vi "FTW-TransferClient-Destroy.vi"(0 "TransferClient.dotNET":refnum<class "FTW-TransferClient-dotNET.lvclass">, 11 "error in":errorcluster) -> (15 "error out":errorcluster)   [LabVIEW 2012, in "FTW-TransferClient-dotNET.lvclass"]
uses:
  FTW-TransferClient-dotNET.lvclass
  FTW-TransferClient.lvclass
  FTW-TransferClient-dotNET.lvclass/FTW-TransferClient-dotNET.ctl
panel:
  # "Inputs"
  # "Outputs"
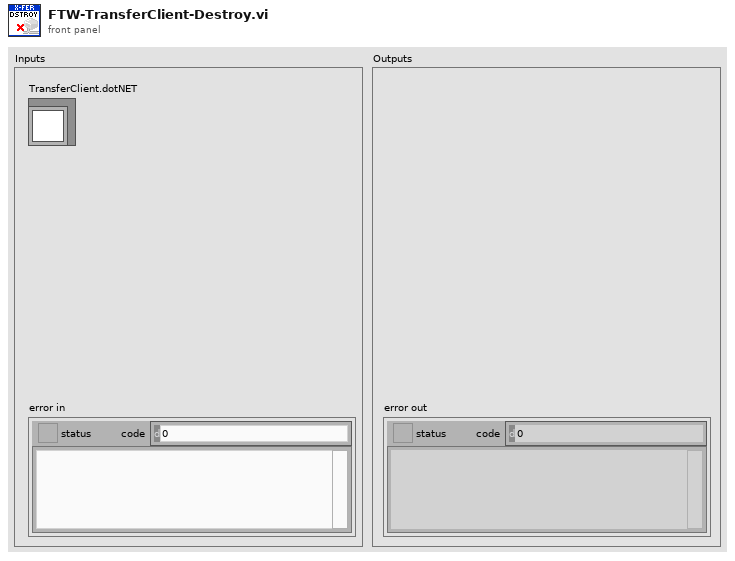
[diagram p1: front panel]
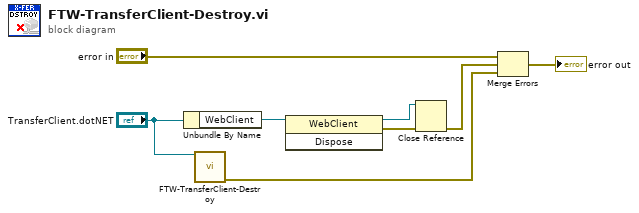
[diagram p0: block diagram]
diagram:
  n1 = Unbundle By Name("TransferClient.dotNET") -> ("WebClient"=w6:refnum<k24>)
  n2 = call-parent "FTW-TransferClient-Destroy.vi"("Transfer Client"="TransferClient.dotNET") -> ("error out"=w1:errorcluster)  [unwired: 14 in]
  n3 = invoke class="WebClient" method="Dispose"(reference=w6) -> (reference out=w5:refnum<k24>, error out=w4:errorcluster)  [unwired: 2 in, 1 out]
  n4 = Close Reference(reference=w5, error in (no error)=w4) -> (error out=w3:errorcluster)
  n5 = Merge Errors("error in", w3, w1) -> (→"error out":errorcluster)
